vi "Drive_V1.vi"(10 "Y_Axis_Right":dbl, 11 "X_Axis_Left":dbl) -> (2 "Numeric 2":dbl, 3 "Numeric":dbl)   [LabVIEW 2013]
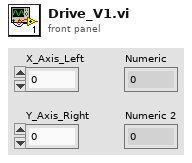
[diagram p1: front panel]
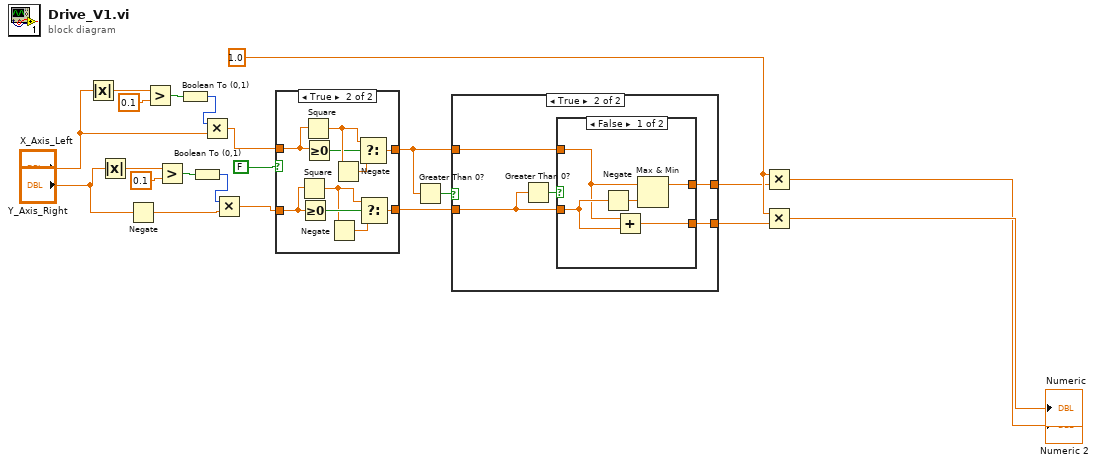
[diagram p0: block diagram]
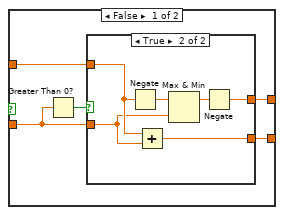
[diagram p2: hidden frame]
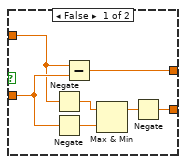
[diagram p3: hidden frame]
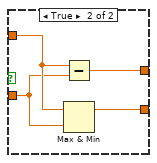
[diagram p4: hidden frame]
diagram:
  w7 = 1.0
  n1 = Absolute Value(x="X_Axis_Left") -> (abs(x)=w11:dbl)
  n2 = Absolute Value(x="Y_Axis_Right") -> (abs(x)=w17:dbl)
  n3 = Negate(x="Y_Axis_Right") -> (-x=w21:dbl)
  n4 = Greater?(x=w11, y=0.1) -> (0:w13:bool)
  n5 = Greater?(x=w17, y=0.1) -> (0:w19:bool)
  n6 = Boolean To (0,1)(Boolean=w13) -> (0, 1=w12:i16)
  n7 = Boolean To (0,1)(Boolean=w19) -> (0, 1=w18:i16)
  n8 = Multiply(x=w12, y="X_Axis_Left") -> (x*y=w15:dbl)
  n9 = Multiply(x=w18, y=w21) -> (x*y=w20:dbl)
  n10 = case shown="True" FALSE {
    tunnel: [w23 w34] -> w3
    tunnel: [w24 w33] -> w2
    tunnel: w20 -> [w23 w32]
    tunnel: w15 -> [w24 w31]
    frame False {
    }
    frame True {
      n11 = Square(x=w32) -> (x^2=w29:dbl)
      n12 = Greater Or Equal To 0?(x=w32) -> (x >= 0?=w30:bool)
      n13 = Square(x=w31) -> (x^2=w26:dbl)
      n14 = Greater Or Equal To 0?(x=w31) -> (x >= 0?=w25:bool)
      n15 = Negate(x=w29) -> (-x=w28:dbl)
      n16 = Negate(x=w26) -> (-x=w27:dbl)
      n17 = Select(t=w26, s=w25, f=w27) -> (s? t:f=w33:dbl)
      n18 = Select(t=w29, s=w30, f=w28) -> (s? t:f=w34:dbl)
    }
  }
  n19 = Greater Than 0?(x=w2) -> (x > 0?=w1:bool)
  n20 = case shown="True" w1 {
    tunnel: w3 -> [w38 w56]
    tunnel: w2 -> [w37 w55]
    tunnel: [w36 w54] -> w4
    tunnel: [w35 w53] -> w5
    frame False {
      n21 = Greater Than 0?(x=w38) -> (x > 0?=w39:bool)
      n22 = case shown="True" w39 {
        tunnel: w38 -> [w46 w48]
        tunnel: w37 -> [w44 w49]
        tunnel: [w40 w50] -> w36
        tunnel: [w41 w47] -> w35
        frame False {
          n23 = Negate(x=w44) -> (-x=w45:dbl)
          n24 = Negate(x=w46) -> (-x=w43:dbl)
          n25 = Subtract(x=w44, y=w46) -> (x-y=w40:dbl)
          n26 = Max & Min(x=w45, y=w43) -> (max(x,y)=w42:dbl)  [unwired: 1 out]
          n27 = Negate(x=w42) -> (-x=w41:dbl)
        }
        frame True {
          n28 = Negate(x=w49) -> (-x=w52:dbl)
          n29 = Add(x=w49, y=w48) -> (x+y=w47:dbl)
          n30 = Max & Min(x=w52, y=w48) -> (max(x,y)=w51:dbl)  [unwired: 1 out]
          n31 = Negate(x=w51) -> (-x=w50:dbl)
        }
      }
    }
    frame True {
      n32 = Greater Than 0?(x=w56) -> (x > 0?=w57:bool)
      n33 = case shown="False" w57 {
        tunnel: w56 -> [w62 w64]
        tunnel: w55 -> [w59 w65]
        tunnel: [w60 w63] -> w54
        tunnel: [w58 w66] -> w53
        frame False {
          n34 = Negate(x=w62) -> (-x=w61:dbl)
          n35 = Add(x=w59, y=w62) -> (x+y=w58:dbl)
          n36 = Max & Min(x=w59, y=w61) -> (max(x,y)=w60:dbl)  [unwired: 1 out]
        }
        frame True {
          n37 = Subtract(x=w65, y=w64) -> (x-y=w63:dbl)
          n38 = Max & Min(x=w65, y=w64) -> (max(x,y)=w66:dbl)  [unwired: 1 out]
        }
      }
    }
  }
  n39 = Multiply(x=w7, y=w4) -> (x*y=→"Numeric 2":dbl)
  n40 = Multiply(x=w7, y=w5) -> (x*y=→"Numeric":dbl)
